vi "Pump Events.vi"(8 "error in":errorcluster) -> (0 "error out":errorcluster)   [LabVIEW 2014, in "LibSDL2.lvlib"]
doc: "Polls for currently pending events.\n\nIf event is not NULL, the next event is removed from the queue and stored in the SDL_Event structure pointed to by event.\n\nAs this function implicitly calls SDL_PumpEvents, you can only call this function in the thread that set the video mode.\n\nReturns 1 if there are any pending events, or 0 if there are none available."
uses:
  LibSDL2.lvlib
  DLL/SDL2.dll
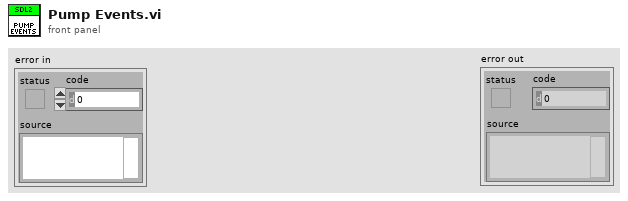
[diagram p1: front panel]
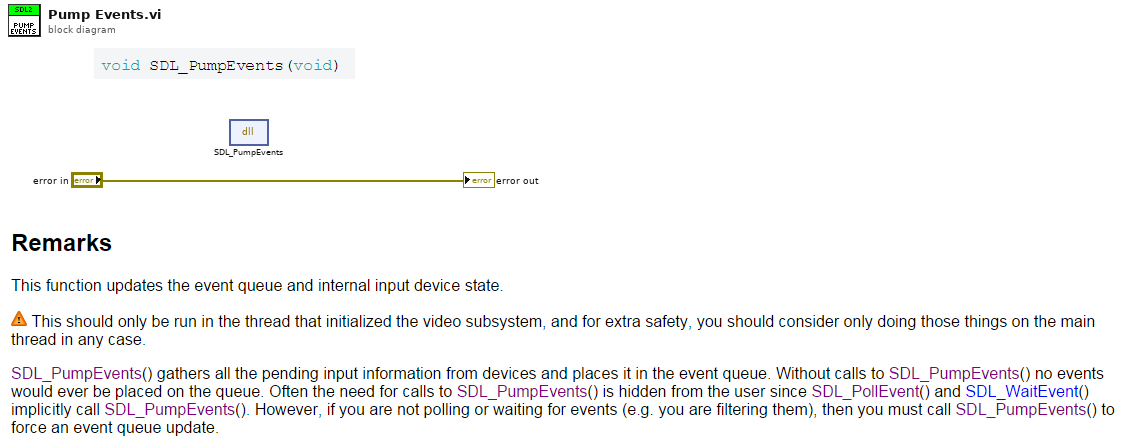
[diagram p0: block diagram]
diagram:
  n1 = dll-call lib="C:/dev/PGS/LabSDL2/Source/Libraries/LibSDL2 Wrapper/DLL/SDL2.dll" fn="SDL_PumpEvents"() -> ()  [unwired: 4 in, 2 out]
  "error out" <- "error in"
